vi "Actor Core.vi"(8 "error in (no error)":errorcluster, 11 "Config GM":refnum<class "Cfg Grandmaster.lvclass">) -> (0 "error out":errorcluster, 3 "Actor Out":refnum<class "Actor.lvclass">)   [LabVIEW 2018, in "Configuration Grandmaster.lvlib" / "Cfg Grandmaster.lvclass"]
uses:
  Cfg Grandmaster.lvclass
  Custom Buttons/Save_Blue.ctl
  Custom Buttons/Open_Blue.ctl
  Custom Buttons/Add_Blue.ctl
  Custom Buttons/Edit_Blue.ctl
  Custom Buttons/Delete_Blue.ctl
  Custom Buttons/New_Blue.ctl
  Custom Buttons/Up_Blue.ctl
  Custom Buttons/Down_Blue.ctl
  Custom Buttons/Wfm_Blue.ctl
  Custom Buttons/Start_Blue.ctl
  Custom Buttons/Stop_Blue.ctl
  Custom Buttons/Refresh_Blue.ctl
  Custom Buttons/Config_Blue.ctl
  Common/Controls/LS Lock Sizes.ctl
  C:/Program Files (x86)/National Instruments/LabVIEW 2018/vi.lib/ActorFramework/Actor/Actor.lvclass
  <vilib>/ActorFramework/Actor/Actor.lvclass
  <vilib>/ActorFramework/Actor/Actor.lvclass/Actor.ctl
  <vilib>/ActorFramework/Message Enqueuer/Message Enqueuer.lvclass/Message Enqueuer.ctl
  Cfg Grandmaster.lvclass/Cfg Grandmaster.ctl
  TCP Server/TCP Writer Messages/Write Data to Stream Msg/Write Data to Conn Msg.lvclass/Write Data to Conn Msg.ctl
  DAQMan Messages/Save Configuration Msg/Save Configuration Msg.lvclass/Save Configuration Msg.ctl
  DAQMan Messages/Load Configuration Msg/Load Configuration Msg.lvclass/Load Configuration Msg.ctl
  Common/Controls/Group Timing Info.ctl
  Common/Controls/TE_Designator.ctl
  DAQMan Messages/Set Timing Msg/Set Timing Msg.lvclass/Set Timing Msg.ctl
  DAQMan Messages/Lock to LS Msg/Lock to LS Msg.lvclass/Lock to LS Msg.ctl
  DAQMan Messages/Set Active Chassis Msg/Set Active Chassis Msg.lvclass/Set Active Chassis Msg.ctl
  Common/Controls/Selected Group.ctl
  DAQMan Messages/Set Selected Group Msg/Set Selected Group Msg.lvclass/Set Selected Group Msg.ctl
  DAQMan Messages/Move Group Position Msg/Move Group Position Msg.lvclass/Move Group Position Msg.ctl
  DAQMan Messages/Add Edit Chan Group Msg/Add Edit Chan Group Msg.lvclass/Add Edit Chan Group Msg.ctl
  Actor Nest/Actor Nest Messages/Handle Nested Error Msg/Handle Nested Error Msg.lvclass/Handle Nested Error Msg.ctl
  <vilib>/ActorFramework/Message Enqueuer/Enqueue.vi
  <vilib>/ActorFramework/Message Enqueuer/Init from Existing Queue.vi
  TCP Server/TCP Writer Messages/Write Data to Stream Msg/Write Data to Conn Msg.lvclass
  C:/Program Files (x86)/National Instruments/LabVIEW 2018/vi.lib/ActorFramework/Message/Message.lvclass
  DAQMan Messages/Clear Config for Active Msg/Clear Config for Active Msg.lvclass
  DAQMan Messages/Save Configuration Msg/Save Configuration Msg.lvclass
  DAQMan Messages/Load Configuration Msg/Load Configuration Msg.lvclass
  DAQMan Messages/Save Workspace Msg/Save Workspace Msg.lvclass
  DAQMan Messages/Set TCP Ports Msg/Set TCP Ports Msg.lvclass
  DAQMan Messages/ShutdownChk Msg/ShutdownChk Msg.lvclass
  DAQMan Messages/Set Timing Msg/Set Timing Msg.lvclass
  DAQMan Messages/Lock to LS Msg/Lock to LS Msg.lvclass
  DAQMan Messages/Set Active Chassis Msg/Set Active Chassis Msg.lvclass
  DAQMan Messages/Initialize DAQMan Msg/Initialize DAQMan Msg.lvclass
  DAQMan Messages/Set Selected Group Msg/Set Selected Group Msg.lvclass
  DAQMan Messages/Move Group Position Msg/Move Group Position Msg.lvclass
  DAQMan Messages/Add Edit Chan Group Msg/Add Edit Chan Group Msg.lvclass
  DAQMan Messages/Delete Chan Group Msg/Delete Chan Group Msg.lvclass
  DAQMan Messages/Configure Chan Group Msg/Configure Chan Group Msg.lvclass
  DAQMan Messages/Stop All DAQ Msg/Stop All DAQ Msg.lvclass
  DAQMan Messages/Start DAQ Msg/Start DAQ Msg.lvclass
  DAQMan Messages/Launch Preview Actor Msg/Launch Preview Actor Msg.lvclass
  Actor Nest/Actor Nest Messages/Handle Nested Error Msg/Handle Nested Error Msg.lvclass
  <vilib>/ActorFramework/Stop Msg/Stop Msg.lvclass
  Common/SubVIs/Conn Status Global.vi
  <vilib>/ActorFramework/Message Priority Queue/Priority Enqueue.vi
  <vilib>/ActorFramework/Message Enqueuer/Message Enqueuer.lvclass
  Actor Nest/Class Actor Nest/Actor Nest.lvclass
panel:
  in  "stop":bool
  out "LS Backlog":dbl(slide) scale=0.0..100.0
  out "HS Backlog":dbl(slide) scale=0.0..100.0
  out "LSGrps Tab":enum32{"GrpList", "AcqCfg"}(tab)
  in  "LS Chan Groups":i32(listbox)=-1
  in  "LS Read Blk":i32=64 caption="Read Block (samps)" step=1
  in  "LS_Cfg":T1
  out "HSGrps Tab":enum32{"GrpList", "AcqCfg"}(tab)
  in  "HS Chan Groups":i32(listbox)=-1
  out "FreqRes":dbl=1.220703125 caption="Frequency Resolution" min=0.0 max=100.0 step=0.1
  in  "HS Read Blk":i32=4096 caption="Read Block (samps)" step=1
  in  "LockToLS":T2 caption="Merge Blocks w/ LS?"
  in  "HS_Cfg":T1
  in  "Mode":string
  in  "Refresh":T3
  in  "Stop":T4
  in  "Start":T5
  in  "Wfm":T6
  in  "LS_Down":T7
  in  "LS_Up":T8
  in  "HS_Down":T7
  in  "HS_Up":T8
  in  "New Cfg":T9
  in  "Delete":T10
  in  "Edit":T11
  in  "Add":T12
  in  "LS Samp Rate":dbl=100.0 caption="Sample Rate" min=0.1 max=1000.0 step=0.1 format="%#_3p"
  in  "HS Samp Rate":dbl=5000.0 min=1000.0 step=0.1 format="%_3p"
  in  "Load Cfg":T13
  in  "Save Cfg":T14
  out "Group Members":i32[](listbox)
  in  "Hardware":string(tree)="cDAQ1"
  out "Runtime Error Count":u32
  out "Rdr Conn":bool
  out "LSConn?":bool
  out "HSConn?":bool
  out "SysTime":string
  # "High Speed"
  # "Low Speed"
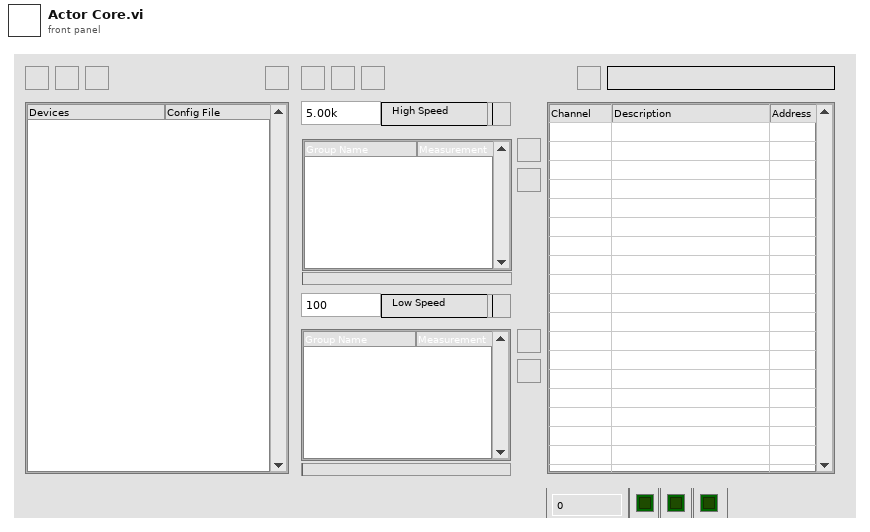
[diagram p1: front panel]
types:
  T1 = typedef "Config_Blue.ctl" = bool
  T2 = typedef "LS Lock Sizes.ctl" = enum16{"No", "250ms", "500ms", "1s"}
  T3 = typedef "Refresh_Blue.ctl" = bool
  T4 = typedef "Stop_Blue.ctl" = bool
  T5 = typedef "Start_Blue.ctl" = bool
  T6 = typedef "Wfm_Blue.ctl" = bool
  T7 = typedef "Down_Blue.ctl" = bool
  T8 = typedef "Up_Blue.ctl" = bool
  T9 = typedef "New_Blue.ctl" = bool
  T10 = typedef "Delete_Blue.ctl" = bool
  T11 = typedef "Edit_Blue.ctl" = bool
  T12 = typedef "Add_Blue.ctl" = bool
  T13 = typedef "Open_Blue.ctl" = bool
  T14 = typedef "Save_Blue.ctl" = bool
  T15 = typedef "TE_Designator.ctl" = enum16{"High Speed", "Low Speed"}
  T16 = typedef "Group Timing Info.ctl" = cluster{"Rate":dbl, "ReadBlk":i32}
  T17 = typedef "Selected Group.ctl" = cluster{"ChanGroup":i32, "Rate Class":T15}
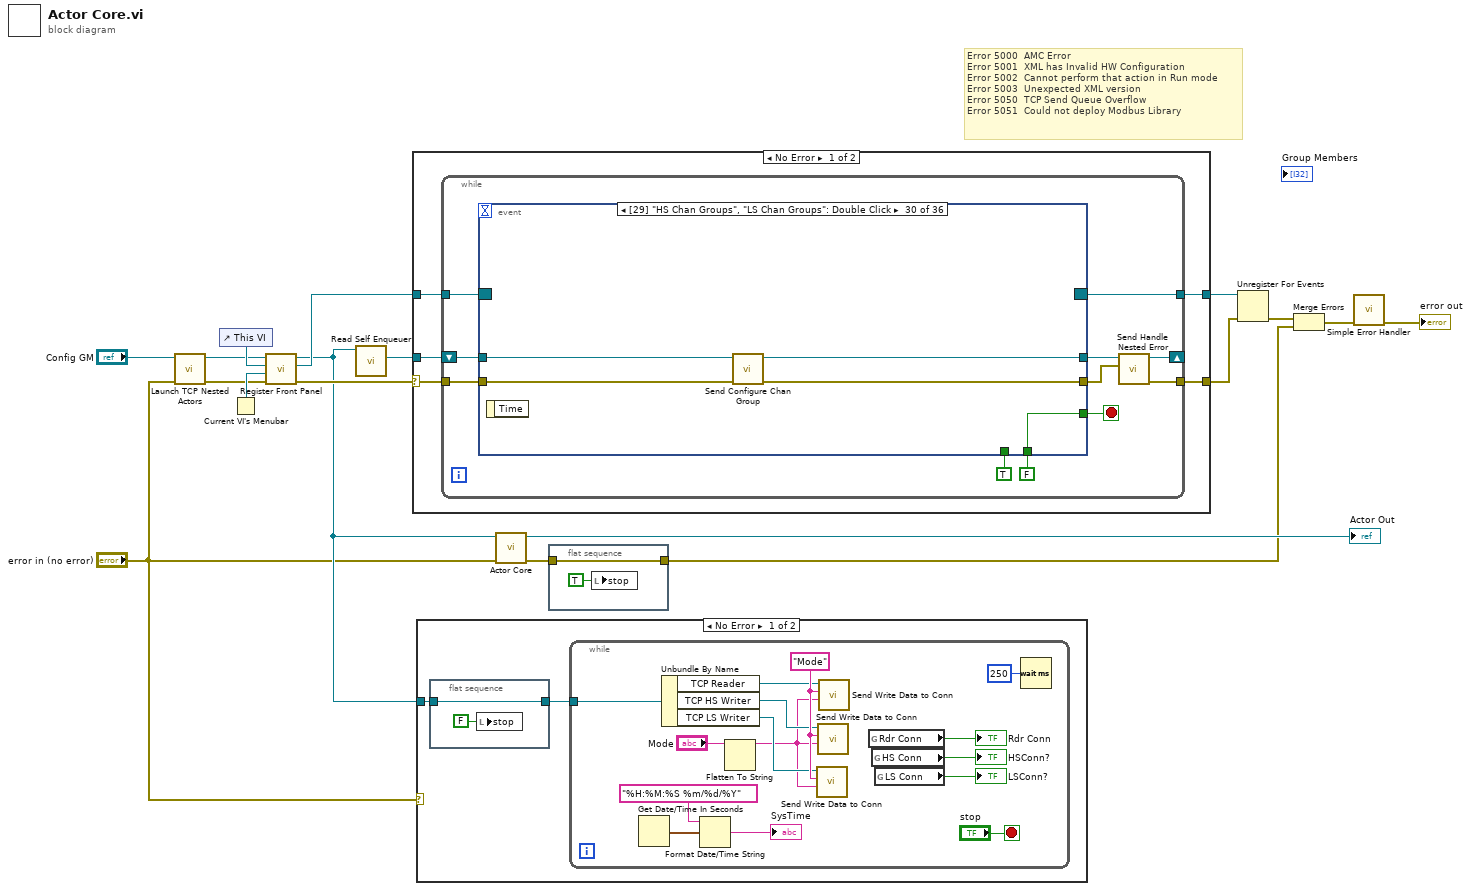
[diagram p0: block diagram]
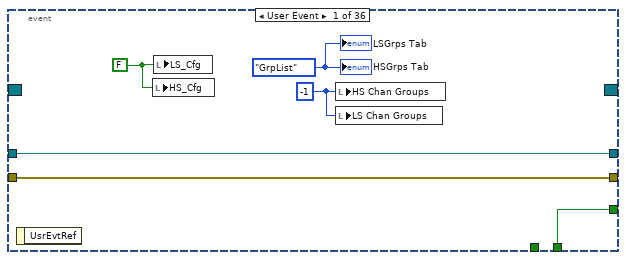
[diagram p3: hidden frame]
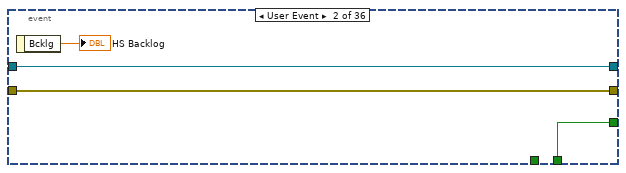
[diagram p4: hidden frame]
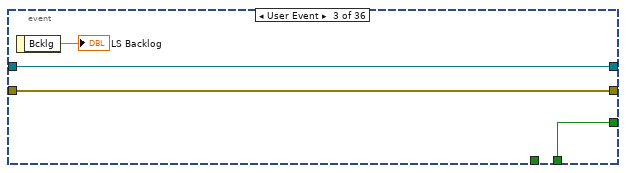
[diagram p5: hidden frame]
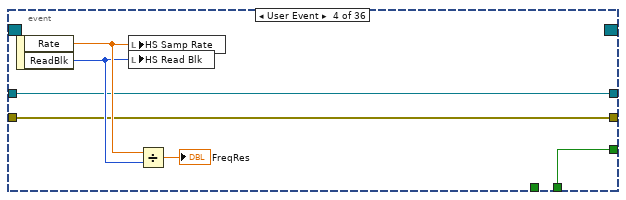
[diagram p6: hidden frame]
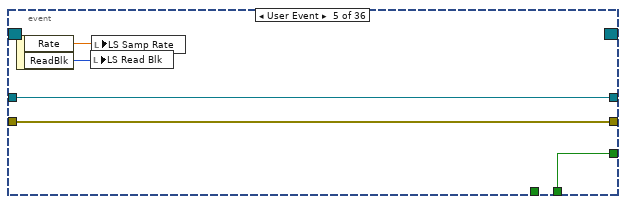
[diagram p7: hidden frame]
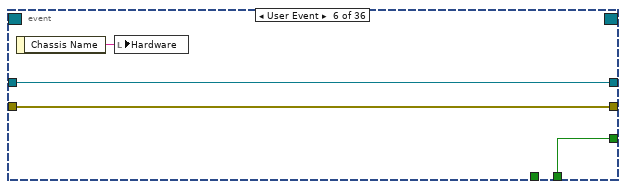
[diagram p8: hidden frame]
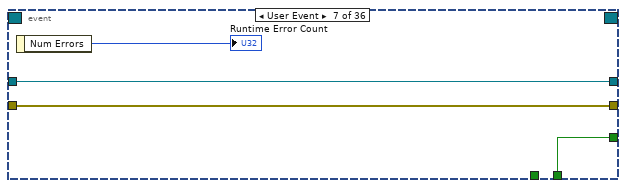
[diagram p9: hidden frame]
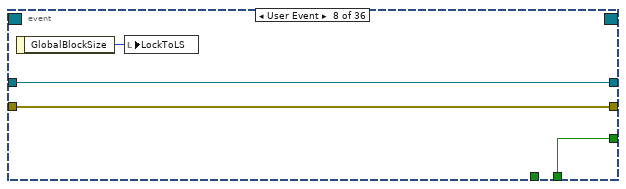
[diagram p10: hidden frame]
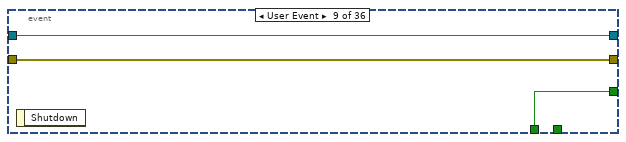
[diagram p11: hidden frame]
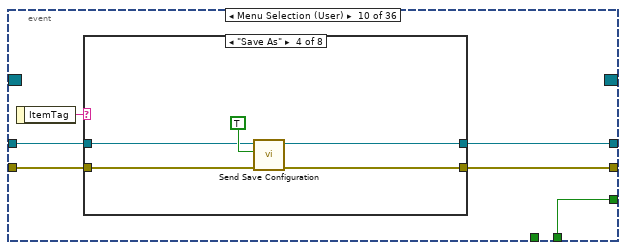
[diagram p12: hidden frame]
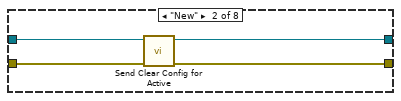
[diagram p14: hidden frame]
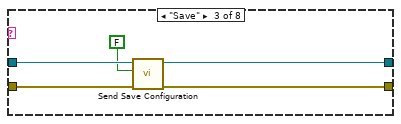
[diagram p15: hidden frame]
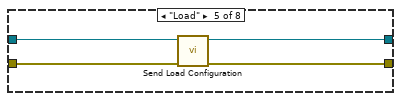
[diagram p16: hidden frame]
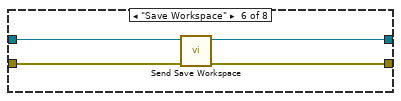
[diagram p17: hidden frame]
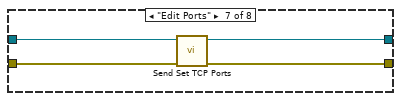
[diagram p18: hidden frame]
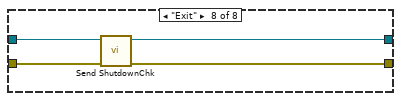
[diagram p19: hidden frame]
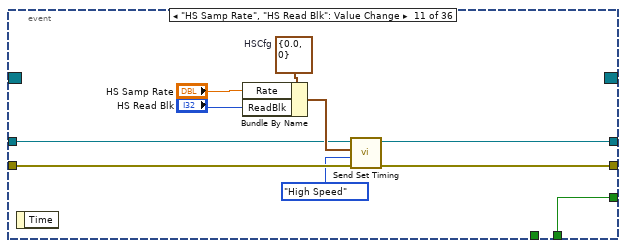
[diagram p20: hidden frame]
diagram:
  # "Error 5000  AMC Error\nError 5001  XML has Invalid HW Configuration\nError 5002  Cannot perform that action in Run mode\nError 5003  Unexpected XML version\nError 5050  TCP Send Queue Overflow\nError 5051  Could not deploy Modbus Library"
  n1 = call-dynamic "Launch TCP Nested Actors.vi"("error in (no error)"="error in (no error)", "Cfg Grandmaster in"="Config GM") -> ("error out"=w8:errorcluster, "Cfg Grandmaster out"=w10:refnum<class "Cfg Grandmaster.lvclass">)  [unwired: 8 in]
  n2 = control-ref of="This VI"() -> (w13:refnum<vi>)
  n3 = Current VI's Menubar() -> (w12:refnum<k9>)
  n4 = call "Register Front Panel.vi"("error in (no error)"=w8, "menu ref"=w12, "This VI"=w13, "DAQMan in"=w10) -> ("error out"=w5:errorcluster, "Event Registration Refnum"=w14:refnum<event-registration>, "DAQMan out"=w2:refnum<class "Cfg Grandmaster.lvclass">)  [unwired: 5 in]
  n5 = call <vilib>:"Read Self Enqueuer.vi"("Actor"=w2) -> ("Self Enqueuer"=w11:refnum<class "Message Enqueuer.lvclass">)  [unwired: 10 in]
  n6 = case shown="No Error" w5 {
    selector: w5 -> [w19 w319]
    tunnel: [w23 w321] -> w18
    tunnel: [w22 w317] -> w17
    tunnel: w14 -> [w21 w321]
    tunnel: w11 -> [w20 w320]
    frame No Error {
      n7 = while {
        tunnel: w19 -> [w34]
        tunnel: w21 -> [w32]
        tunnel: [w30] -> w23
        tunnel: [w27] -> w22
        shift-right: [w24] -> _
        shift-left: w20 -> [w26]
        stop <- w33 stop-if-true
        n8 = event shown="[29] \"HS Chan Groups\", \"LS Chan Groups\": Double Click" {
          selector: w32 -> [_ _ _ _ _ _ _ _ _ _ _ _ _ _ _ _ _ _ _ _ _ _ _ _ _ _ _ _ _ _ _ _ _ _ _ _]
          dyn-events: [_ _ _ _ _ _ _ _ _ _ _ _ _ _ _ _ _ _ _ _ _ _ _ _ _ _ _ _ _ _ _ _ _ _ _ _] -> w30
          timeout: _ -> [_ _ _ _ _ _ _ _ _ _ _ _ _ _ _ _ _ _ _ _ _ _ _ _ _ _ _ _ _ _ _ _ _ _ _ _]
          tunnel: w34 -> [w38 w44 w48 w51 w59 w62 w66 w70 w73 w79 w116 w127 w137 w143 w148 w154 w161 w168 w173 w178 w183 w193 w205 w220 w234 w248 w259 w266 w271 w276 w281 w286 w291 w296 w305 w313]
          tunnel: [w38 w44 w48 w51 w59 w62 w66 w70 w73 w80 w118 w128 w136 w142 w147 w153 w161 w168 w172 w177 w182 w194 w206 w217 w229 w243 w258 w265 w270 w275 w280 w285 w290 w295 w303 w314] -> w28
          tunnel: [w37 w43 w45 w50 w58 w61 w65 w68 w74 w77 w121 w129 w138 w144 w149 w155 w162 w169 w174 w179 w185 w195 w203 w219 w233 w247 w261 w267 w272 w277 w282 w287 w292 w297 w306 w315] -> w33
          tunnel: TRUE ("stop") -> [_ _ _ _ _ _ _ _ w74 _ _ _ _ _ _ _ _ _ _ _ _ _ _ _ _ _ _ _ _ _ _ _ _ _ _ w316]
          tunnel: FALSE ("stop") -> [w37 w43 w45 w50 w58 w61 w65 w68 _ w77 w121 w129 w138 w144 w149 w155 w162 w169 w174 w179 w185 w195 w203 w219 w233 w247 w261 w267 w272 w277 w282 w287 w292 w297 w306 w315]
          tunnel: w26 -> [w35 w42 w47 w49 w55 w60 w67 w69 w72 w76 w115 w125 w134 w140 w146 w152 w156 w163 w171 w176 w181 w192 w201 w216 w232 w244 w260 w264 w269 w274 w279 w284 w289 w293 w302 w312]
          tunnel: [w35 w42 w47 w49 w55 w60 w67 w69 w72 w75 w113 w123 w133 w139 w145 w150 w156 w163 w170 w175 w180 w190 w200 w214 w228 w242 w256 w262 w268 w273 w278 w283 w288 w293 w302 w311] -> w25
          event User Event {
            w40 = -1 ("HS Chan Groups")
            w39 = T1 FALSE ("HS_Cfg")
            w36 = enum32{"GrpList", "AcqCfg"}."GrpList" ("HSGrps Tab")
            n9 = event-data() -> ()  [unwired: 1 in, 1 out]
            n10 = local write "HS_Cfg"(w39) -> ()
            n11 = local write "LS_Cfg"(w39) -> ()
            n12 = local write "HS Chan Groups"(w40) -> ()
            n13 = local write "LS Chan Groups"(w40) -> ()
            "LSGrps Tab" <- w36
            "HSGrps Tab" <- w36
          }
          event User Event {
            n14 = event-data() -> ("Bcklg"=→"HS Backlog":dbl)  [unwired: 1 in]
          }
          event User Event {
            n15 = event-data() -> ("Bcklg"=→"LS Backlog":dbl)  [unwired: 1 in]
          }
          event User Event {
            n16 = event-data() -> ("Rate"=w53:dbl, "ReadBlk"=w52:i32)  [unwired: 1 in]
            n17 = local write "HS Samp Rate"(w53) -> ()
            n18 = local write "HS Read Blk"(w52) -> ()
            n19 = Divide(x=w53, y=w52) -> (x/y=→"FreqRes":dbl)
          }
          event User Event {
            n20 = event-data() -> ("Rate"=w57:dbl, "ReadBlk"=w56:i32)  [unwired: 1 in]
            n21 = local write "LS Read Blk"(w56) -> ()
            n22 = local write "LS Samp Rate"(w57) -> ()
          }
          event User Event {
            n23 = event-data() -> ("Chassis Name"=w63:string)  [unwired: 1 in]
            n24 = local write "Hardware"(w63) -> ()
          }
          event User Event {
            n25 = event-data() -> ("Num Errors"=→"Runtime Error Count":u32)  [unwired: 1 in]
          }
          event User Event {
            n26 = event-data() -> ("GlobalBlockSize"=w71:T2)  [unwired: 1 in]
            n27 = local write "LockToLS"(w71) -> ()
          }
          event User Event {
            n28 = event-data() -> ()  [unwired: 1 in, 1 out]
          }
          event Menu Selection (User) {
            n29 = event-data() -> ("ItemTag"=w78:string)  [unwired: 1 in]
            n30 = case shown="\"Save As\"" w78 {
              tunnel: [w82 w85 w90 w94 w100 w104 w108 w111] -> w80
              tunnel: w79 -> [w82 w86 w91 w95 w99 w103 w107 w112]
              tunnel: w76 -> [w81 w84 w89 w93 w98 w102 w106 w110]
              tunnel: [w81 w83 w87 w92 w97 w101 w105 w109] -> w75
              frame Default {
              }
              frame "New" {
                n31 = call "Send Clear Config for Active.vi"("error in (no error)"=w86, "Message Enqueuer"=w84) -> ("error out"=w85:errorcluster, "Message Enqueuer out"=w83:refnum<class "Message Enqueuer.lvclass">)  [unwired: 8 in]
              }
              frame "Save" {
                n32 = call "Send Save Configuration.vi"("error in (no error)"=w91, "Save As?"=FALSE, "Message Enqueuer"=w89) -> ("error out"=w90:errorcluster, "Message Enqueuer out"=w87:refnum<class "Message Enqueuer.lvclass">)  [unwired: 7 in]
              }
              frame "Save As" {
                n33 = call "Send Save Configuration.vi"("error in (no error)"=w95, "Save As?"=TRUE, "Message Enqueuer"=w93) -> ("error out"=w94:errorcluster, "Message Enqueuer out"=w92:refnum<class "Message Enqueuer.lvclass">)  [unwired: 7 in]
              }
              frame "Load" {
                n34 = call "Send Load Configuration.vi"("error in (no error)"=w99, "Message Enqueuer"=w98) -> ("error out"=w100:errorcluster, "Message Enqueuer out"=w97:refnum<class "Message Enqueuer.lvclass">)  [unwired: 8 in]
              }
              frame "Save Workspace" {
                n35 = call "Send Save Workspace.vi"("error in (no error)"=w103, "Message Enqueuer"=w102) -> ("error out"=w104:errorcluster, "Message Enqueuer out"=w101:refnum<class "Message Enqueuer.lvclass">)  [unwired: 8 in]
              }
              frame "Edit Ports" {
                n36 = call "Send Set TCP Ports.vi"("error in (no error)"=w107, "Message Enqueuer"=w106) -> ("error out"=w108:errorcluster, "Message Enqueuer out"=w105:refnum<class "Message Enqueuer.lvclass">)  [unwired: 8 in]
              }
              frame "Exit" {
                n37 = call "Send ShutdownChk.vi"("error in (no error)"=w112, "Message Enqueuer"=w110) -> ("error out"=w111:errorcluster, "Message Enqueuer out"=w109:refnum<class "Message Enqueuer.lvclass">)  [unwired: 8 in]
              }
            }
          }
          event "HS Samp Rate", "HS Read Blk": Value Change {
            w119 = T16 {"Rate"=0.0, "ReadBlk"=0}  # HSCfg
            n38 = event-data() -> ()  [unwired: 1 in, 1 out]
            n39 = Bundle By Name(cluster=w119, "Rate"="HS Samp Rate", "ReadBlk"="HS Read Blk") -> (w117:T16)
            n40 = call "Send Set Timing.vi"("error in (no error)"=w116, "Timing Engine"=TE_Designator."High Speed", "Timing Info"=w117, "Message Enqueuer"=w115) -> ("error out"=w118:errorcluster, "Message Enqueuer out"=w113:refnum<class "Message Enqueuer.lvclass">)  [unwired: 6 in]
          }
          event "LS Samp Rate", "LS Read Blk": Value Change {
            w132 = T16 {"Rate"=0.0, "ReadBlk"=0}  # HSCfg
            n41 = event-data() -> ()  [unwired: 1 in, 1 out]
            n42 = Bundle By Name(cluster=w132, "Rate"="LS Samp Rate", "ReadBlk"="LS Read Blk") -> (w126:T16)
            n43 = call "Send Set Timing.vi"("error in (no error)"=w127, "Timing Engine"=TE_Designator."Low Speed", "Timing Info"=w126, "Message Enqueuer"=w125) -> ("error out"=w128:errorcluster, "Message Enqueuer out"=w123:refnum<class "Message Enqueuer.lvclass">)  [unwired: 6 in]
          }
          event Value Change {
            n44 = event-data() -> ()  [unwired: 1 in, 1 out]
            n45 = call "Send Lock to LS.vi"("error in (no error)"=w137, "LockToLS"="LockToLS", "Message Enqueuer"=w134) -> ("error out"=w136:errorcluster, "Message Enqueuer out"=w133:refnum<class "Message Enqueuer.lvclass">)  [unwired: 7 in]
          }
          event "Hardware": Value Change {
            n46 = event-data() -> ()  [unwired: 1 in, 1 out]
            n47 = call "Send Set Active Chassis.vi"("error in (no error)"=w143, "Chassis Name"="Hardware", "Message Enqueuer"=w140) -> ("error out"=w142:errorcluster, "Message Enqueuer out"=w139:refnum<class "Message Enqueuer.lvclass">)  [unwired: 7 in]
          }
          event Value Change {
            n48 = event-data() -> ()  [unwired: 1 in, 1 out]
            n49 = call "Send Clear Config for Active.vi"("error in (no error)"=w148, "Message Enqueuer"=w146) -> ("error out"=w147:errorcluster, "Message Enqueuer out"=w145:refnum<class "Message Enqueuer.lvclass">)  [unwired: 8 in]
          }
          event Value Change {
            n50 = event-data() -> ()  [unwired: 1 in, 1 out]
            n51 = call "Send Save Configuration.vi"("error in (no error)"=w154, "Save As?"=FALSE, "Message Enqueuer"=w152) -> ("error out"=w153:errorcluster, "Message Enqueuer out"=w150:refnum<class "Message Enqueuer.lvclass">)  [unwired: 7 in]
          }
          event Value Change {
            n52 = event-data() -> ()  [unwired: 1 in, 3 out]
            n53 = Select(t=enum32{"GrpList", "AcqCfg"}."AcqCfg" ("HSGrps Tab"), s="HS_Cfg", f=enum32{"GrpList", "AcqCfg"}."GrpList" ("HSGrps Tab")) -> (s? t:f=w157:enum32{"GrpList", "AcqCfg"})
            n54 = local write "HSGrps Tab"(w157) -> ()
          }
          event Value Change {
            n55 = event-data() -> ()  [unwired: 1 in, 3 out]
            n56 = Select(t=enum32{"GrpList", "AcqCfg"}."AcqCfg" ("HSGrps Tab"), s="LS_Cfg", f=enum32{"GrpList", "AcqCfg"}."GrpList" ("HSGrps Tab")) -> (s? t:f=w167:enum32{"GrpList", "AcqCfg"})
            n57 = local write "LSGrps Tab"(w167) -> ()
          }
          event Value Change {
            n58 = event-data() -> ()  [unwired: 1 in, 1 out]
            n59 = call "Send Load Configuration.vi"("error in (no error)"=w173, "Message Enqueuer"=w171) -> ("error out"=w172:errorcluster, "Message Enqueuer out"=w170:refnum<class "Message Enqueuer.lvclass">)  [unwired: 8 in]
          }
          event Value Change {
            n60 = event-data() -> ()  [unwired: 1 in, 1 out]
            n61 = call "Send Initialize DAQMan.vi"("error in (no error)"=w178, "Message Enqueuer"=w176) -> ("error out"=w177:errorcluster, "Message Enqueuer out"=w175:refnum<class "Message Enqueuer.lvclass">)  [unwired: 8 in]
          }
          event "HS Chan Groups": Value Change {
            w188 = T17 {"ChanGroup"=0, "Rate Class"=enum."High Speed"}  # Selected Group
            n62 = event-data() -> ()  [unwired: 1 in, 1 out]
            n63 = Bundle By Name(cluster=w188, "ChanGroup"="HS Chan Groups", "Rate Class"=TE_Designator."High Speed") -> (w184:T17)
            n64 = call "Send Set Selected Group.vi"("error in (no error)"=w183, "Selected Group"=w184, "Message Enqueuer"=w181) -> ("error out"=w182:errorcluster, "Message Enqueuer out"=w180:refnum<class "Message Enqueuer.lvclass">)  [unwired: 7 in]
            n65 = local write "LS Chan Groups"(-1 ("LS Chan Groups")) -> ()
          }
          event "LS Chan Groups": Value Change {
            w198 = T17 {"ChanGroup"=0, "Rate Class"=enum."High Speed"}  # Selected Group
            n66 = event-data() -> ()  [unwired: 1 in, 1 out]
            n67 = Bundle By Name(cluster=w198, "ChanGroup"="LS Chan Groups", "Rate Class"=TE_Designator."Low Speed") -> (w191:T17)
            n68 = call "Send Set Selected Group.vi"("error in (no error)"=w193, "Selected Group"=w191, "Message Enqueuer"=w192) -> ("error out"=w194:errorcluster, "Message Enqueuer out"=w190:refnum<class "Message Enqueuer.lvclass">)  [unwired: 7 in]
            n69 = local write "HS Chan Groups"(-1 ("HS Chan Groups")) -> ()
          }
          event Value Change {
            n70 = event-data() -> ()  [unwired: 1 in, 1 out]
            n71 = property on="HS Chan Groups" class="MCListbox (strict)"(error in=w205) -> (error out=w204:errorcluster, "Value"=w202:i32)  [unwired: 1 in, 1 out]
            n72 = case shown="Default" w202 {
              tunnel: [w208 w212] -> w206
              tunnel: w204 -> [w208 w213]
              tunnel: w201 -> [w207 w211]
              tunnel: [w207 w209] -> w200
              frame -1 {
              }
              frame Default {
                n73 = call "Send Move Group Position.vi"("error in (no error)"=w213, "Up (T) / Down (F)"=TRUE, "Message Enqueuer"=w211) -> ("error out"=w212:errorcluster, "Message Enqueuer out"=w209:refnum<class "Message Enqueuer.lvclass">)  [unwired: 7 in]
              }
            }
          }
          event Value Change {
            n74 = event-data() -> ()  [unwired: 1 in, 1 out]
            n75 = property on="HS Chan Groups" class="MCListbox (strict)"(error in=w220) -> (error out=w218:errorcluster, "Value"=w215:i32)  [unwired: 1 in, 1 out]
            n76 = case shown="Default" w215 {
              tunnel: [w222 w226] -> w217
              tunnel: w218 -> [w222 w227]
              tunnel: w216 -> [w221 w225]
              tunnel: [w221 w223] -> w214
              frame -1 {
              }
              frame Default {
                n77 = call "Send Move Group Position.vi"("error in (no error)"=w227, "Up (T) / Down (F)"=FALSE, "Message Enqueuer"=w225) -> ("error out"=w226:errorcluster, "Message Enqueuer out"=w223:refnum<class "Message Enqueuer.lvclass">)  [unwired: 7 in]
              }
            }
          }
          event Value Change {
            n78 = event-data() -> ()  [unwired: 1 in, 1 out]
            n79 = property on="LS Chan Groups" class="MCListbox (strict)"(error in=w234) -> (error out=w231:errorcluster, "Value"=w230:i32)  [unwired: 1 in, 1 out]
            n80 = case shown="Default" w230 {
              tunnel: [w236 w240] -> w229
              tunnel: w231 -> [w236 w241]
              tunnel: w232 -> [w235 w239]
              tunnel: [w235 w237] -> w228
              frame -1 {
              }
              frame Default {
                n81 = call "Send Move Group Position.vi"("error in (no error)"=w241, "Up (T) / Down (F)"=TRUE, "Message Enqueuer"=w239) -> ("error out"=w240:errorcluster, "Message Enqueuer out"=w237:refnum<class "Message Enqueuer.lvclass">)  [unwired: 7 in]
              }
            }
          }
          event Value Change {
            n82 = event-data() -> ()  [unwired: 1 in, 1 out]
            n83 = property on="LS Chan Groups" class="MCListbox (strict)"(error in=w248) -> (error out=w246:errorcluster, "Value"=w245:i32)  [unwired: 1 in, 1 out]
            n84 = case shown="Default" w245 {
              tunnel: [w250 w254] -> w243
              tunnel: w246 -> [w250 w255]
              tunnel: w244 -> [w249 w253]
              tunnel: [w249 w251] -> w242
              frame -1 {
              }
              frame Default {
                n85 = call "Send Move Group Position.vi"("error in (no error)"=w255, "Up (T) / Down (F)"=FALSE, "Message Enqueuer"=w253) -> ("error out"=w254:errorcluster, "Message Enqueuer out"=w251:refnum<class "Message Enqueuer.lvclass">)  [unwired: 7 in]
              }
            }
          }
          event Value Change {
            n86 = event-data() -> ()  [unwired: 1 in, 1 out]
            n87 = call "Send Add Edit Chan Group.vi"("error in (no error)"=w259, "Add (F) / Edit (T)"=FALSE, "Message Enqueuer"=w260) -> ("error out"=w258:errorcluster, "Message Enqueuer out"=w256:refnum<class "Message Enqueuer.lvclass">)  [unwired: 7 in]
          }
          event Value Change {
            n88 = event-data() -> ()  [unwired: 1 in, 1 out]
            n89 = call "Send Add Edit Chan Group.vi"("error in (no error)"=w266, "Add (F) / Edit (T)"=TRUE, "Message Enqueuer"=w264) -> ("error out"=w265:errorcluster, "Message Enqueuer out"=w262:refnum<class "Message Enqueuer.lvclass">)  [unwired: 7 in]
          }
          event Value Change {
            n90 = event-data() -> ()  [unwired: 1 in, 1 out]
            n91 = call "Send Delete Chan Group.vi"("error in (no error)"=w271, "Message Enqueuer"=w269) -> ("error out"=w270:errorcluster, "Message Enqueuer out"=w268:refnum<class "Message Enqueuer.lvclass">)  [unwired: 8 in]
          }
          event "HS Chan Groups", "LS Chan Groups": Double Click {
            n92 = event-data() -> ()  [unwired: 1 in, 1 out]
            n93 = call "Send Configure Chan Group.vi"("error in (no error)"=w276, "Message Enqueuer"=w274) -> ("error out"=w275:errorcluster, "Message Enqueuer out"=w273:refnum<class "Message Enqueuer.lvclass">)  [unwired: 8 in]
          }
          event Value Change {
            n94 = event-data() -> ()  [unwired: 1 in, 1 out]
            n95 = call "Send Stop All DAQ.vi"("error in (no error)"=w281, "Message Enqueuer"=w279) -> ("error out"=w280:errorcluster, "Message Enqueuer out"=w278:refnum<class "Message Enqueuer.lvclass">)  [unwired: 8 in]
          }
          event Value Change {
            n96 = event-data() -> ()  [unwired: 1 in, 1 out]
            n97 = call "Send Start DAQ.vi"("error in (no error)"=w286, "Message Enqueuer"=w284) -> ("error out"=w285:errorcluster, "Message Enqueuer out"=w283:refnum<class "Message Enqueuer.lvclass">)  [unwired: 8 in]
          }
          event Value Change {
            n98 = event-data() -> ()  [unwired: 1 in, 1 out]
            n99 = call "Send Launch Preview Actor.vi"("error in (no error)"=w291, "Message Enqueuer"=w289) -> ("error out"=w290:errorcluster, "Message Enqueuer out"=w288:refnum<class "Message Enqueuer.lvclass">)  [unwired: 8 in]
          }
          event "HS Backlog": Mouse Enter {
            n100 = event-data() -> ()  [unwired: 1 in, 2 out]
            n101 = local read "HS Backlog"() -> (w301:dbl)
            n102 = Number To Fractional String(number=w301, precision (6)=i16 1) -> (F-format string=w299:string)  [unwired: 2 in]
            n103 = Concatenate Strings(w299, "% Buffer Backlog" ("string")) -> (w294:string)
            n104 = property on="HS Backlog" class="Slide (strict)"(error in=w296, "TipStrip"=w294) -> (error out=w295:errorcluster)  [unwired: 1 in, 1 out]
          }
          event "LS Backlog": Mouse Enter {
            n105 = event-data() -> ()  [unwired: 1 in, 1 out]
            n106 = local read "LS Backlog"() -> (w310:dbl)
            n107 = Number To Fractional String(number=w310, precision (6)=i16 1) -> (F-format string=w308:string)  [unwired: 2 in]
            n108 = Concatenate Strings(w308, "% Buffer Backlog" ("string")) -> (w304:string)
            n109 = property on="LS Backlog" class="Slide (strict)"(error in=w305, "TipStrip"=w304) -> (error out=w303:errorcluster)  [unwired: 1 in, 1 out]
          }
          event Panel Close? {
            n110 = event-data() -> ()  [unwired: 1 in, 1 out]
            n111 = call "Send ShutdownChk.vi"("error in (no error)"=w313, "Message Enqueuer"=w312) -> ("error out"=w314:errorcluster, "Message Enqueuer out"=w311:refnum<class "Message Enqueuer.lvclass">)  [unwired: 8 in]
            n112 = event-data("Discard?"=w316) -> ()  [unwired: 1 in, 1 out]
          }
        }
        n113 = call "Send Handle Nested Error.vi"("Nested Error"=w28, "Message Enqueuer"=w25) -> ("error out"=w27:errorcluster, "Message Enqueuer out"=w24:refnum<class "Message Enqueuer.lvclass">)  [unwired: 8 in]
      }
    }
    frame Error {
      n114 = call "Send Handle Nested Error.vi"("Nested Error"=w319, "Message Enqueuer"=w320) -> ("Message Enqueuer out"=w318:refnum<class "Message Enqueuer.lvclass">)  [unwired: 8 in, 1 out]
      n115 = call <vilib>:"Send Normal Stop.vi"("Message Enqueuer"=w318) -> ("error out"=w317:errorcluster)  [unwired: 10 in]
    }
  }
  n116 = case shown="No Error" "error in (no error)" {
    tunnel: w2 -> [w322 _]
    frame No Error {
      n117 = flat-sequence {
        tunnel: [w339] -> w323
        tunnel: w322 -> [w339]
        frame #0 {
          n118 = local write "stop"(FALSE ("stop")) -> ()
        }
      }
      n119 = while {
        tunnel: w323 -> [w329]
        stop <- "stop" stop-if-true
        w338 = "Mode" ("MetaData")
        n120 = Get Date/Time In Seconds() -> (seconds since 1Jan1904=w328:timestamp)
        n121 = Unbundle By Name(w329) -> ("TCP Reader"=w331:refnum<class "Message Enqueuer.lvclass">, "TCP HS Writer"=w336:refnum<class "Message Enqueuer.lvclass">, "TCP LS Writer"=w337:refnum<class "Message Enqueuer.lvclass">)
        n122 = Format Date/Time String(time format string (%c)="%H:%M:%S %m/%d/%Y", seconds (now)=w328) -> (date/time string=→"SysTime":string)  [unwired: 1 in]
        n123 = Flatten To String(anything="Mode") -> (data string=w326:string)  [unwired: 3 in, 2 out]
        n124 = call "Send Write Data to Conn.vi"("Data"=w326, "MetaData"=w338, "Message Enqueuer"=w337) -> ()  [unwired: 7 in, 2 out]
        n125 = call "Send Write Data to Conn.vi"("Data"=w326, "MetaData"=w338, "Message Enqueuer"=w336) -> ()  [unwired: 7 in, 2 out]
        n126 = call "Send Write Data to Conn.vi"("Data"=w326, "MetaData"=w338, "Message Enqueuer"=w331) -> ()  [unwired: 7 in, 2 out]
        n127 = global read "Conn Status Global.vi" "Rdr Conn"() -> (→"Rdr Conn":bool)
        n128 = global read "Conn Status Global.vi" "HS Conn"() -> (→"HSConn?":bool)
        n129 = global read "Conn Status Global.vi" "LS Conn"() -> (→"LSConn?":bool)
        n130 = Wait (ms)(milliseconds to wait=u32 250) -> ()  [unwired: 1 out]
      }
    }
    frame Error {
    }
  }
  n131 = call-parent "Actor Core.vi"("error in"="error in (no error)", "Actor in"=w2) -> ("error out"=w4:errorcluster, "Actor out"=→"Actor Out":refnum<class "Actor.lvclass">)  [unwired: 8 in]
  n132 = flat-sequence {
    tunnel: w4 -> [w342]
    tunnel: [w342] -> w3
    frame #0 {
      n133 = local write "stop"(TRUE ("stop")) -> ()
    }
  }
  n134 = Unregister For Events(event registration refnum=w18, error in=w17) -> (error out=w15:errorcluster)
  n135 = Merge Errors(w15, w3) -> (w7:errorcluster)
  n136 = call <vilib>:"Simple Error Handler.vi"("error in (no error)"=w7) -> ("error out"=→"error out":errorcluster)  [unwired: 4 in, 4 out]
